vi "DAQ Input Handler.vi"(8 "error in (no error)":errorcluster, 11 "Message Queues out":T1) -> (0 "error out":errorcluster, 3 "Message Queue":refnum<queue>)   [LabVIEW 2014]
uses:
  support/Message Queue/All Message Queues.ctl
  support/Message Queue/Message Cluster.ctl
  Teszt/Teszt.ctl
  Teszt/Command.ctl
  Engine/Message.ctl
  Digital/Digital Input Cluster.ctl
  Digital/Digital Output Cluster.ctl
  <vilib>/Analysis/baseanly.llb/Mean (DBL).vi
  support/Message Queue/Enqueue Message (Single).vi
  <vilib>/Utility/error.llb/Error Cluster From Error Code.vi
  <vilib>/ErrorRing/Error Ring.xnode
  support/Message Queue/Message Queue.lvlib
  <vilib>/Analysis/NI_AALBase.lvlib
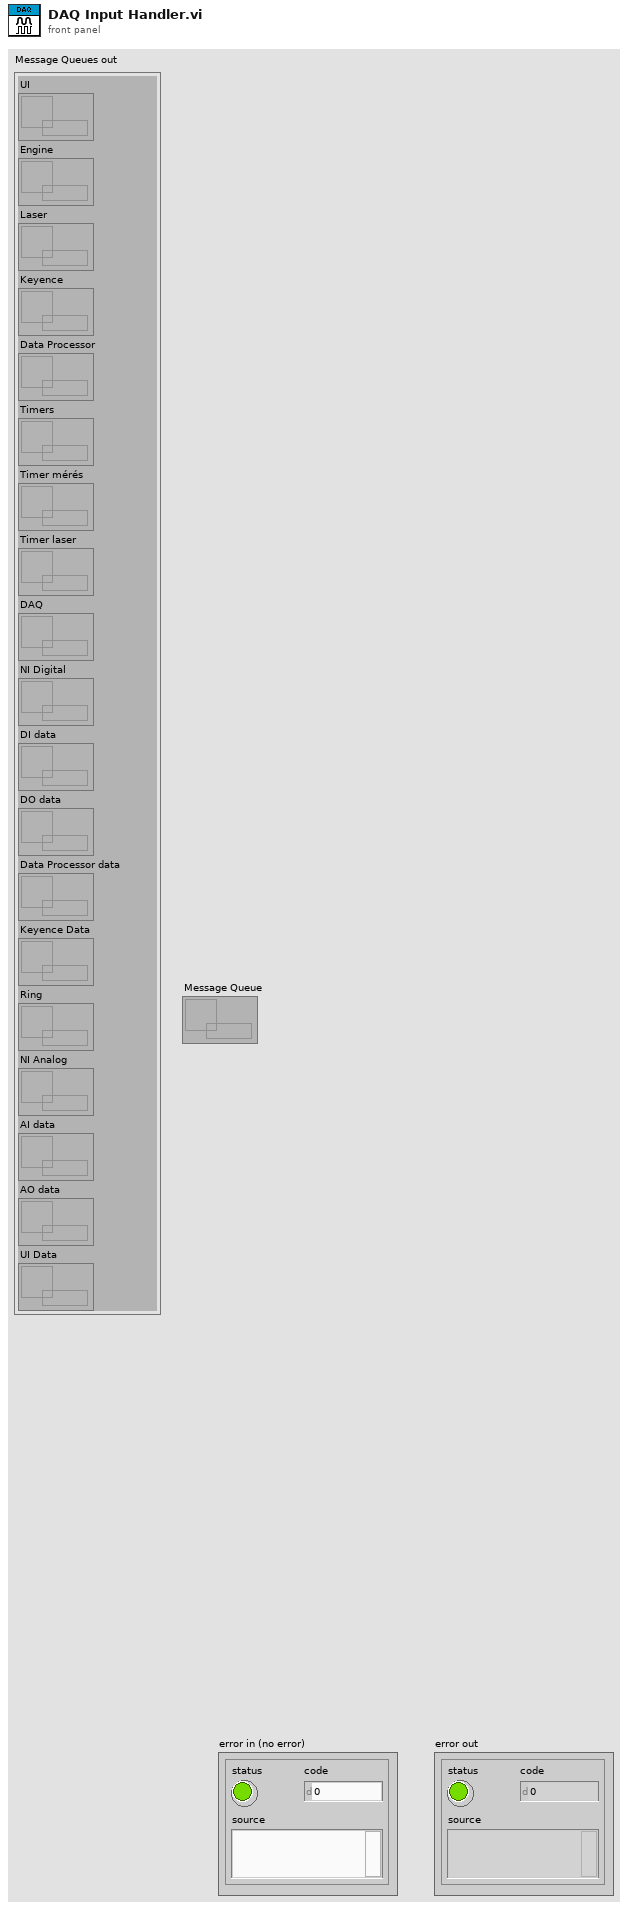
[diagram p1: front panel]
types:
  T1 = typedef "Message Queue.lvlib/All Message Queues.ctl" = cluster{"UI":refnum<queue>, "Engine":refnum<queue>, "Laser":refnum<queue>, "Keyence":refnum<queue>, "Data Processor":refnum<queue>, "Timers":refnum<queue>, "Timer mérés":refnum<queue>, "Timer laser":refnum<queue>, "DAQ":refnum<queue>, "NI Digital":refnum<queue>, "DI data":refnum<queue>, "DO data":refnum<queue>, "Data Processor data":refnum<queue>, "Keyence Data":refnum<queue>, "Ring":refnum<queue>, "NI Analog":refnum<queue>, "AI data":refnum<queue>, "AO data":refnum<queue>, "UI Data":refnum<queue>}
  T2 = typedef "Digital Output Cluster.ctl" = cluster{"PCIE-6321 OUT":cluster{"Izolációs relé":bool, "B oldal relé (nincs használva)":bool, "48V relé":bool, "Elszívás KI":bool, "Bördelezés teszt":bool, "Gyûrû megnyomás":bool, "Termék rögzítés":bool, "R mérés relé":bool, "200mA relé":bool, "NTC mérés relé":bool, "Levegõ BE":bool}}
  T3 = typedef "Digital Input Cluster.ctl" = cluster{"PCIE-6321 IN":cluster{"Termék bördelezve":bool, "Izolációs relék OK":bool, "Rézgyûrû a terméken":bool, "Termék rögzítve":bool, "Termék a gyûrûzõben":bool, "Rézgyûrû behelyezve":bool, "Rézgyûrû elengedve":bool, "Rézgyûrû megnyomva":bool, "Termék elengedve":bool, "Levegõ rendben":bool, "Termék jelen (táv)":bool, "Termék jelen (fém)":bool, "Selejt érzékelõ":bool}}
  T4 = typedef "Message.ctl" = cluster{"Thread ID":u16, "Callback":string, "Data":variant, "Error":errorcluster}
  T5 = typedef "Teszt.ctl" = cluster{"Thread ID":dbl, "Mérésszám":string, "Mérés/Utasítás":string, "Command":T6, "Min":string, "Max":string, "Aktív?":bool, "Log?":bool, "Kiértékelés":bool, "Etalon 1 exp":bool, "Etalon 2 exp":bool, "Etalon 3 exp":bool, "Etalon 4 exp":bool, "Etalon 5 exp":bool}
  T6 = typedef "Command.ctl" = cluster{"Parancs":string, "Paraméter 1":string, "Paraméter 2":string, "Paraméter 3":string, "Paraméter 4":string, "Paraméter 5":string, "Eredmény":string}
  T7 = cluster{"Termék bördelezve":bool, "Izolációs relék OK":bool, "Rézgyûrû a terméken":bool, "Termék rögzítve":bool, "Termék a gyûrûzõben":bool, "Rézgyûrû behelyezve":bool, "Rézgyûrû elengedve":bool, "Rézgyûrû megnyomva":bool, "Termék elengedve":bool, "Levegõ rendben":bool, "Termék jelen (táv)":bool, "Termék jelen (fém)":bool, "Selejt érzékelõ":bool}
  T8 = cluster{"Izolációs relé":bool, "B oldal relé (nincs használva)":bool, "48V relé":bool, "Elszívás KI":bool, "Bördelezés teszt":bool, "Gyûrû megnyomás":bool, "Termék rögzítés":bool, "R mérés relé":bool, "200mA relé":bool, "NTC mérés relé":bool, "Levegõ BE":bool}
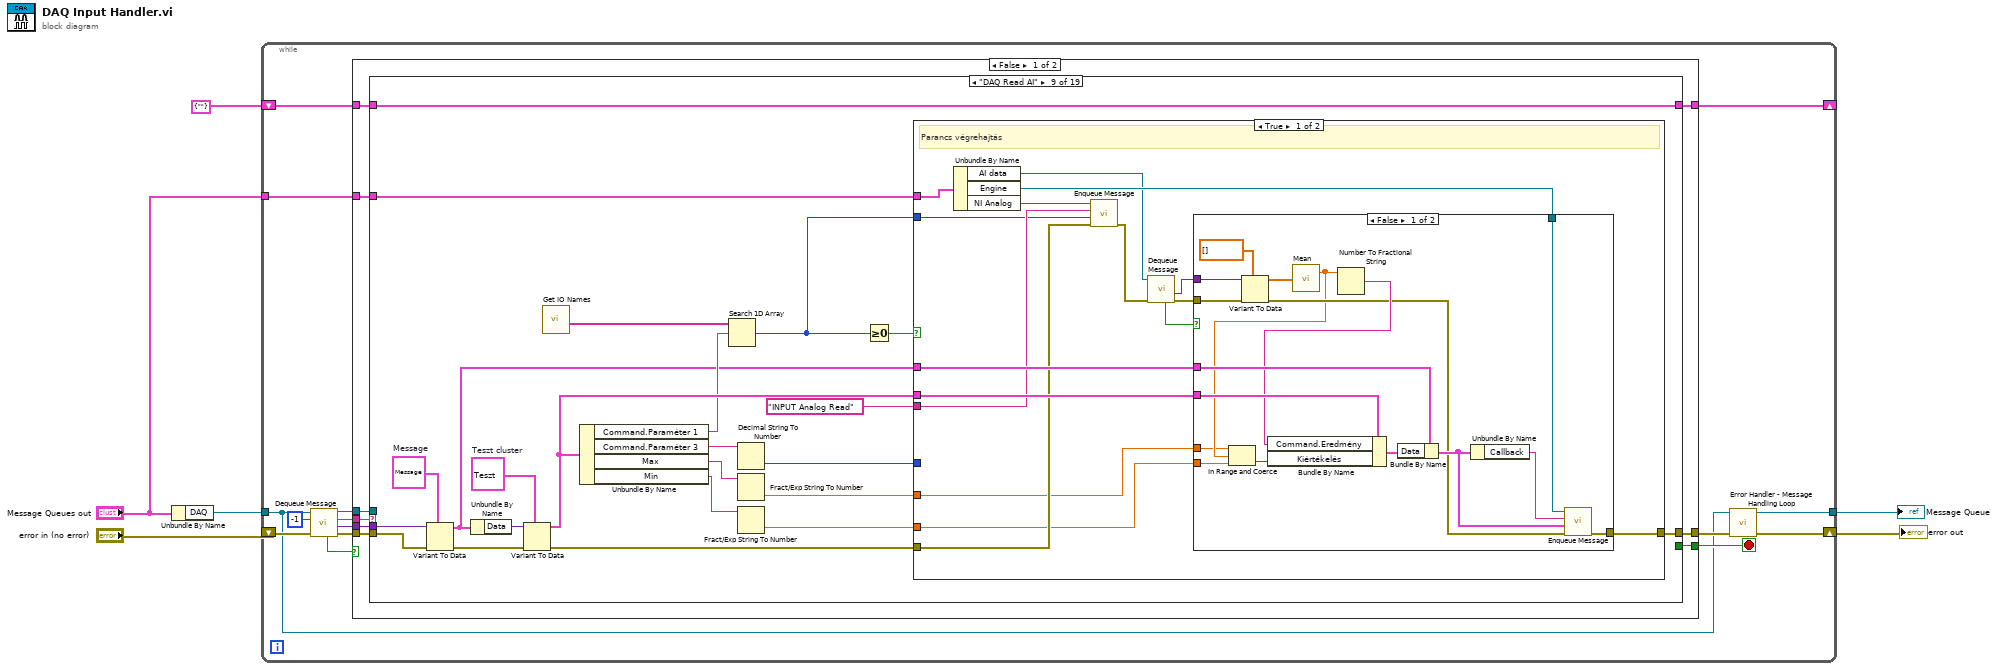
[diagram p0: block diagram]
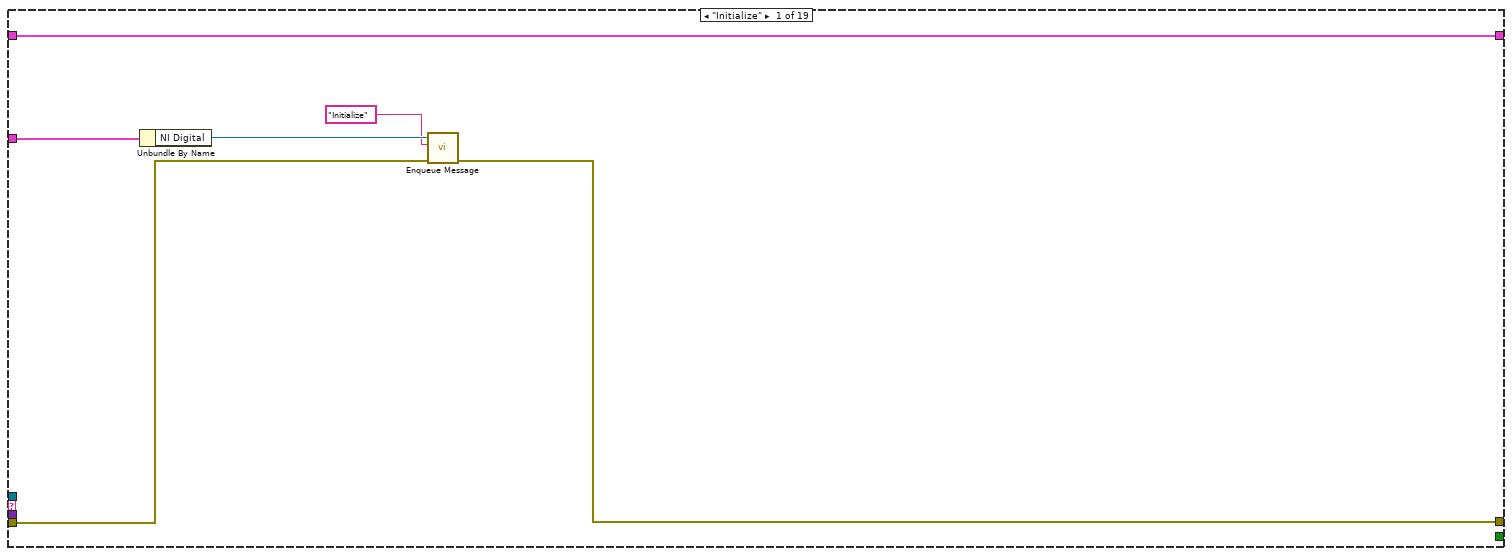
[diagram p2: hidden frame]
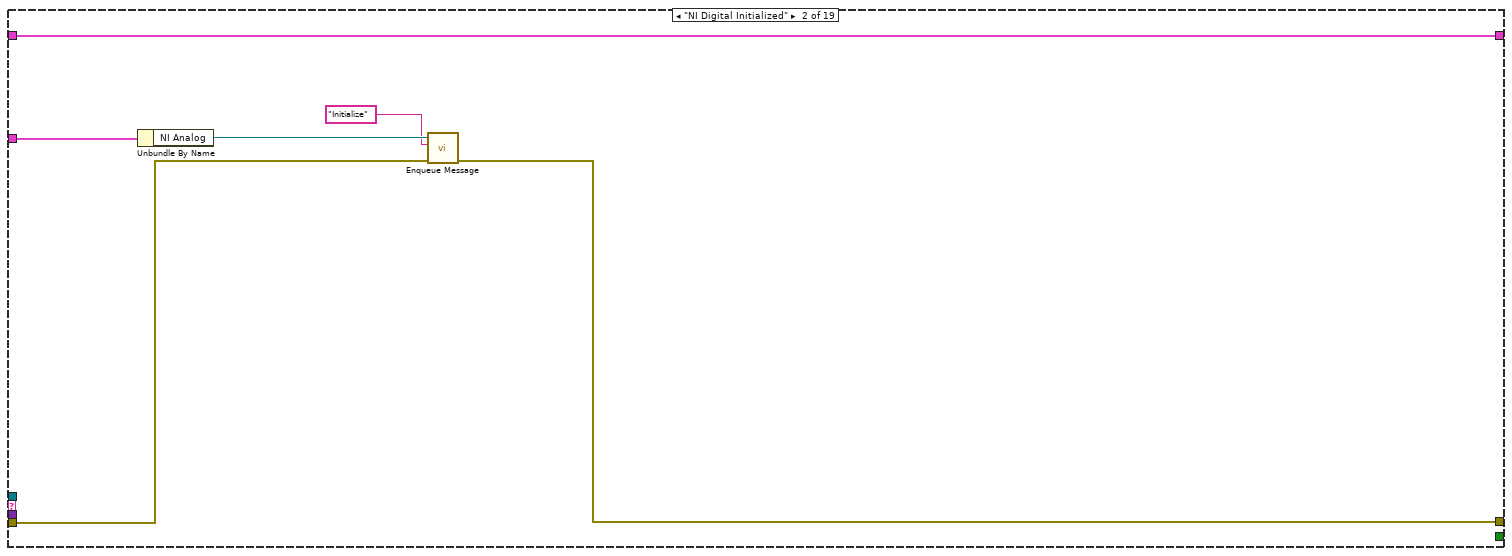
[diagram p3: hidden frame]
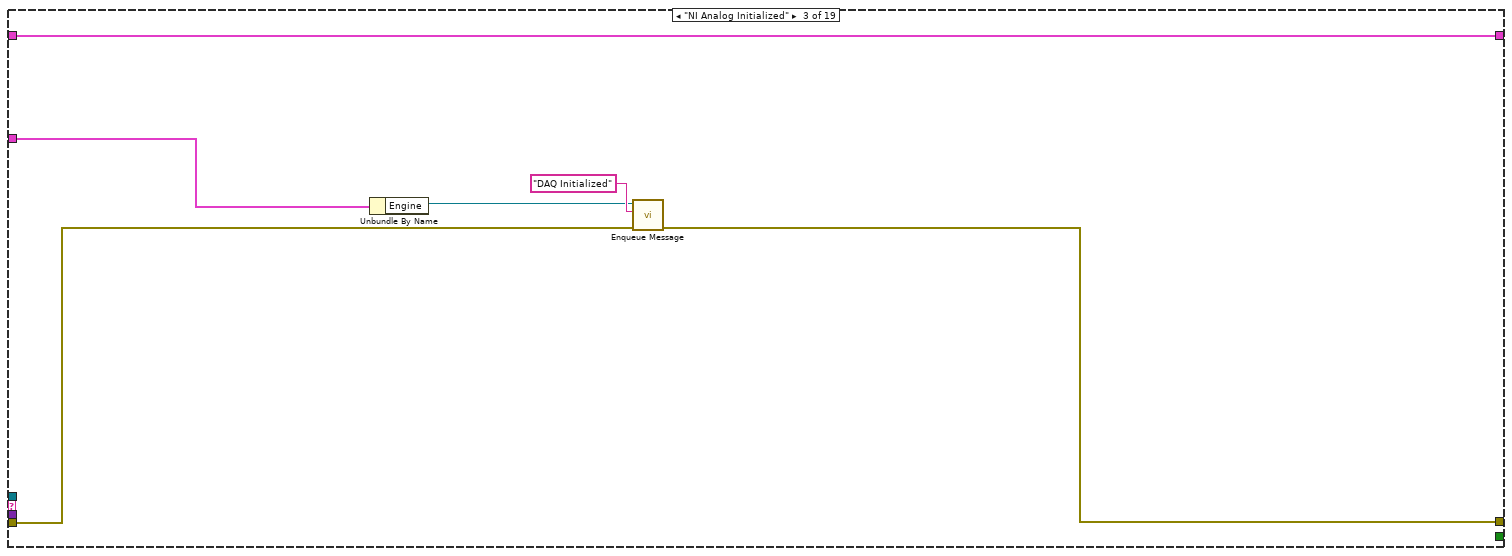
[diagram p4: hidden frame]
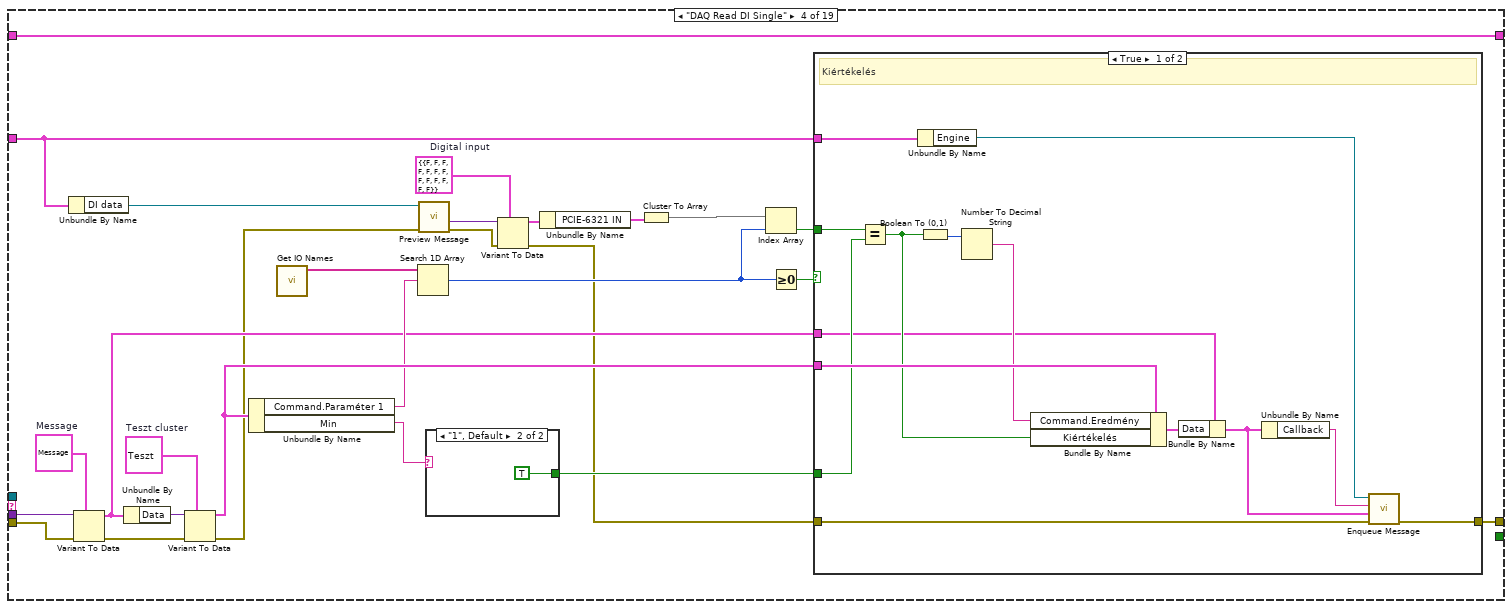
[diagram p5: hidden frame]
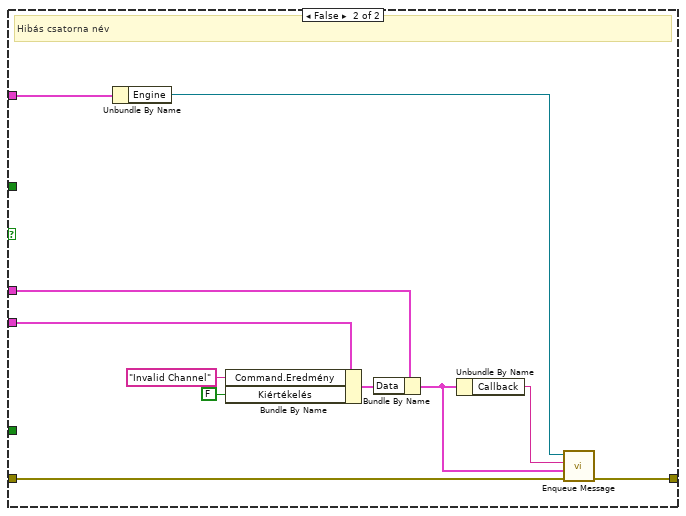
[diagram p6: hidden frame]
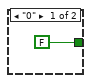
[diagram p7: hidden frame]
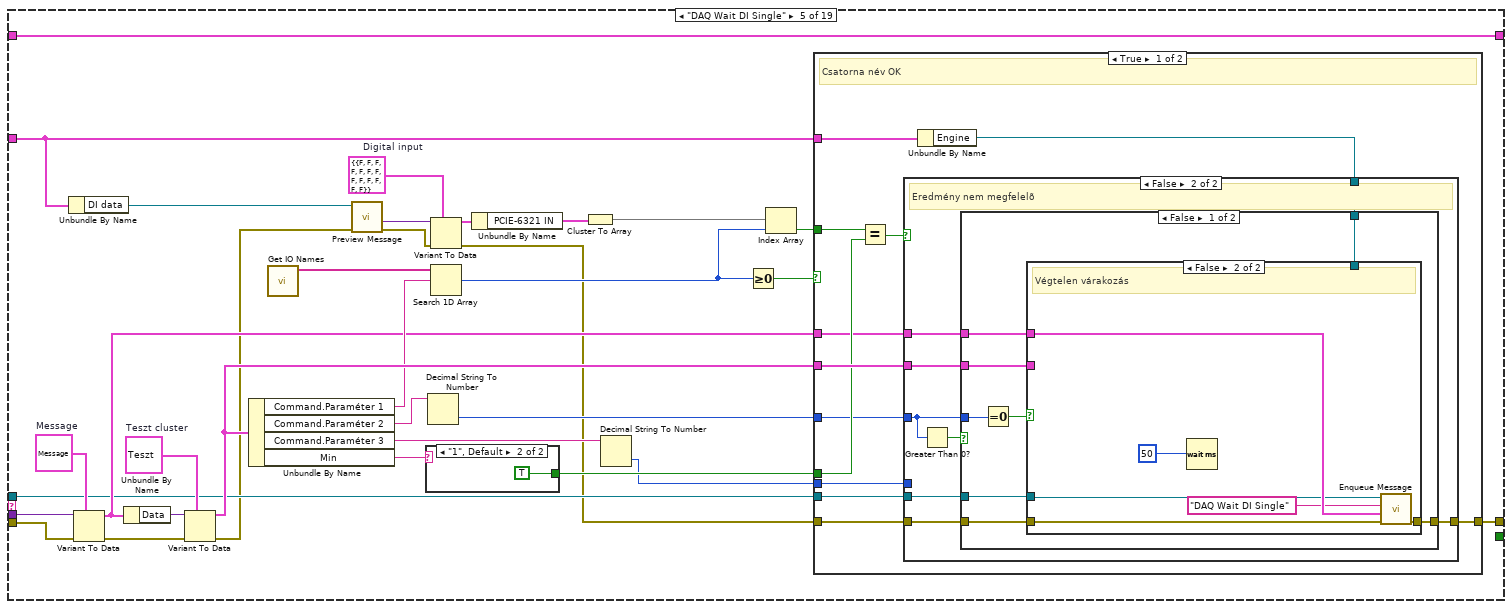
[diagram p8: hidden frame]
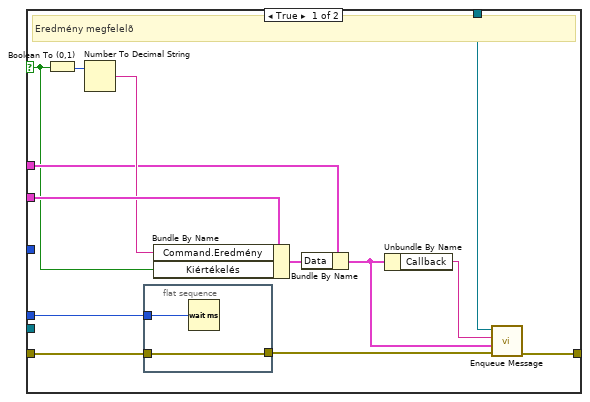
[diagram p9: hidden frame]
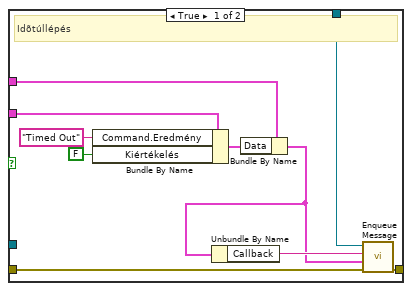
[diagram p10: hidden frame]
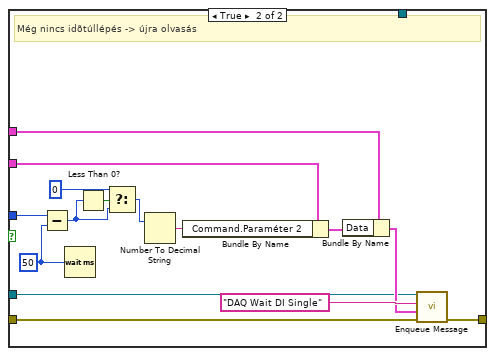
[diagram p11: hidden frame]
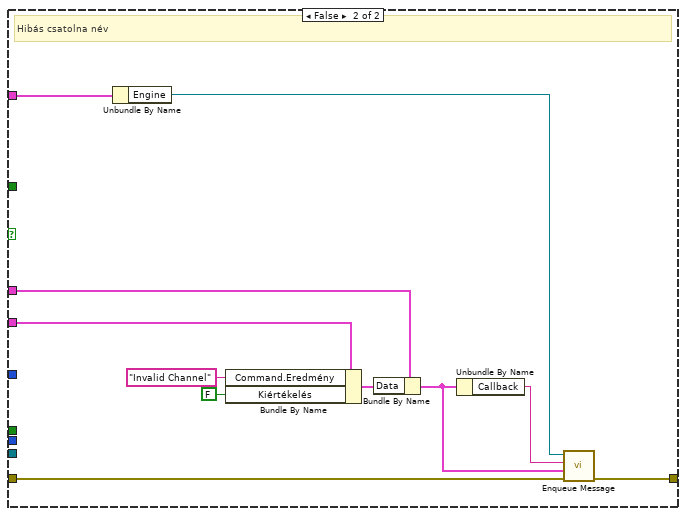
[diagram p12: hidden frame]
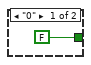
[diagram p13: hidden frame]
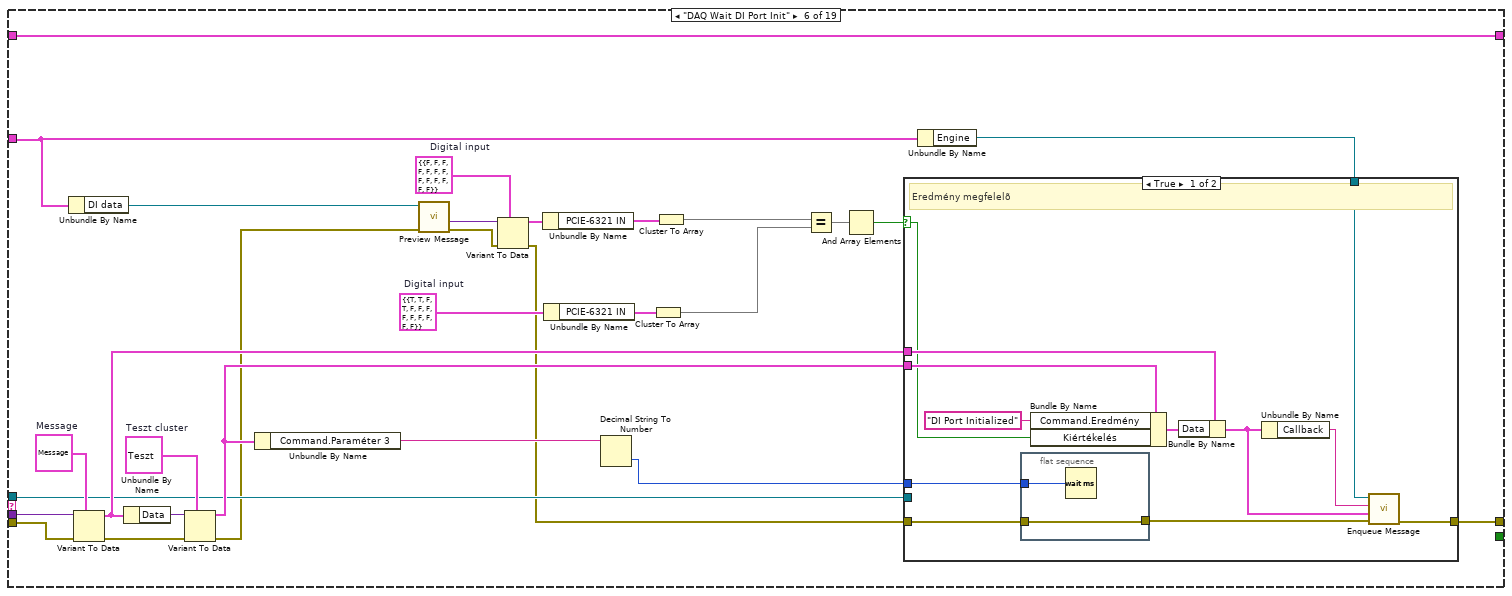
[diagram p14: hidden frame]
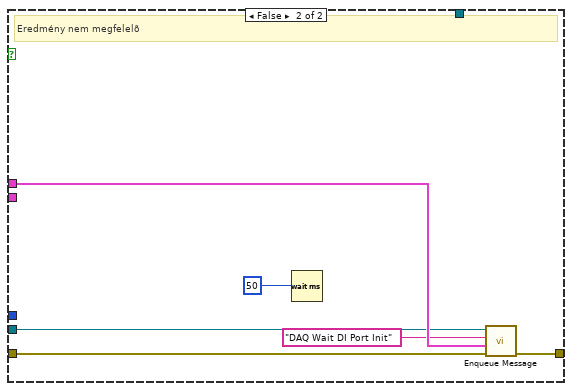
[diagram p15: hidden frame]
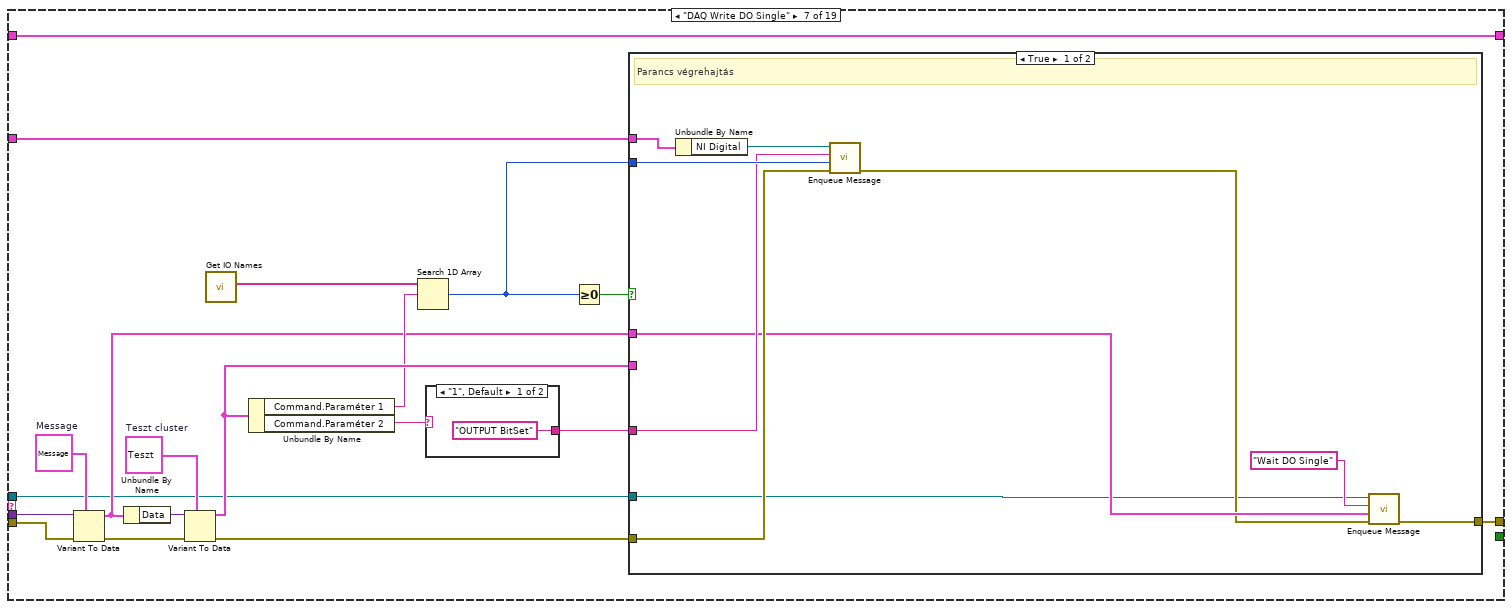
[diagram p16: hidden frame]
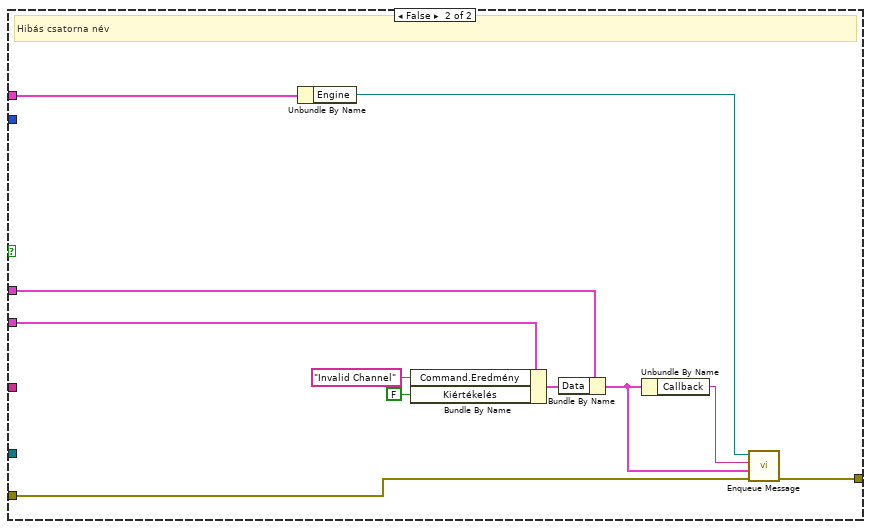
[diagram p17: hidden frame]
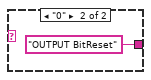
[diagram p18: hidden frame]
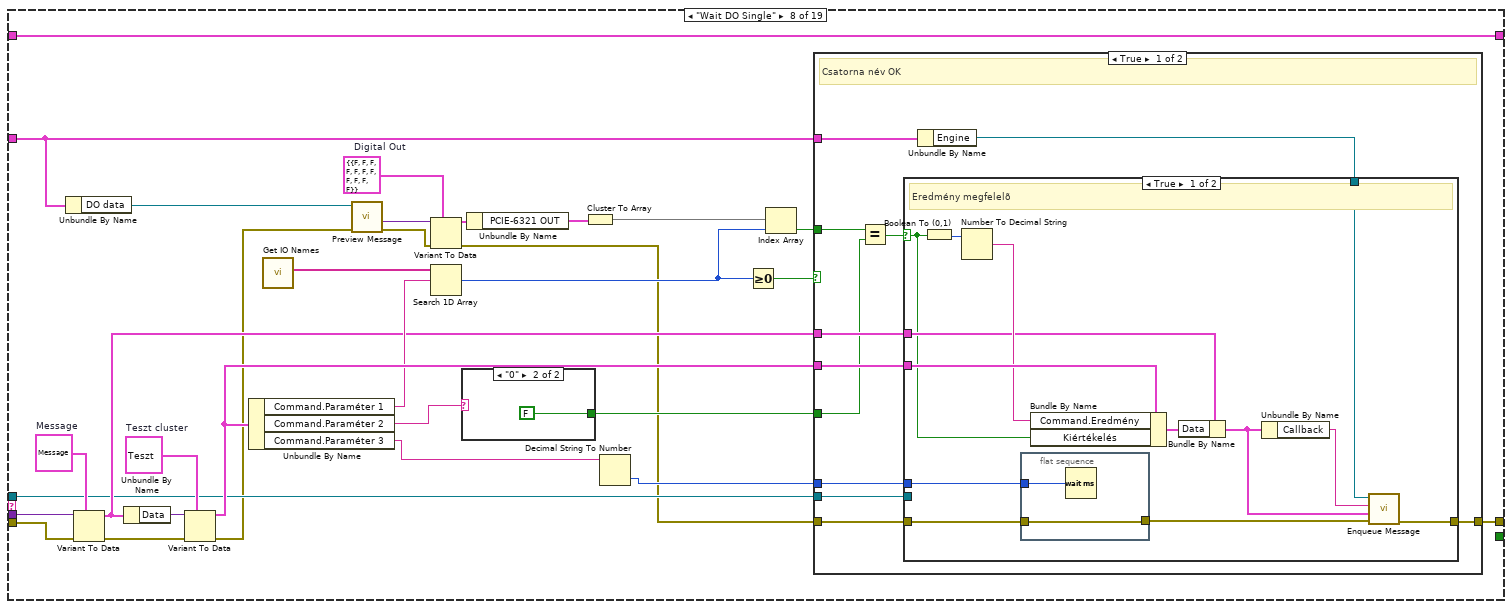
[diagram p19: hidden frame]
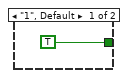
[diagram p20: hidden frame]
diagram:
  n1 = Unbundle By Name("Message Queues out") -> ("DAQ"=w3:refnum<queue>)
  n2 = while {
    tunnel: w3 -> [w7]
    shift-right: [w13] -> w6
    shift-left: "error in (no error)" -> [w21]
    tunnel: "Message Queues out" -> [w11]
    tunnel: [w10] -> w4
    shift-right: [w8] -> _
    shift-left: cluster{"Enabled Connectors":string} {"Enabled Connectors"=""} -> [w9]
    stop <- w17 stop-if-true
    n3 = call "Dequeue Message.vi"("error in (no error)"=w21, "timeout in ms (-1)"=-1, "Message Queue"=w7) -> ("error out"=w19:errorcluster, "Message Data"=w14:variant, "Message"=w20:string, "dup Message Queue"=w18:refnum<queue>, "timed out?"=w15:bool)  [unwired: 4 in]
    n4 = case shown="False" w15 {
      tunnel: w20 -> [w30 _]
      tunnel: w19 -> [w29 w655]
      tunnel: w18 -> [w28 _]
      tunnel: [w27 FALSE] -> w17
      tunnel: [w26 w655] -> w12
      tunnel: w14 -> [w25 _]
      tunnel: w11 -> [w24 _]
      tunnel: w9 -> [w23 w653]
      tunnel: [w22 w653] -> w8
      frame False {
        n5 = case shown="\"DAQ Read AI\"" w30 {
          selector: w30 -> [_ _ _ _ _ _ _ _ _ _ _ _ _ _ _ _ _ _ w643]
          tunnel: w29 -> [w33 w39 w44 w71 w130 w246 w284 w338 w405 w481 w538 w568 w587 w608 w619 w624 w633 w642 _]
          tunnel: w28 -> [_ _ _ _ w107 w234 w271 w319 _ _ _ _ _ _ w618 w631 w636 w641 _]
          tunnel: [w32 w38 w48 w70 w129 w245 w283 w337 w404 w480 w537 w567 w586 w607 w617 w621 w637 w639 w644] -> w26
          tunnel: [_ _ _ _ _ _ _ _ _ _ _ _ _ _ _ _ _ TRUE _] -> w27
          tunnel: w25 -> [_ _ _ w68 w127 w243 w281 w335 w402 w478 w535 w565 w585 w606 _ w625 _ _ _]
          tunnel: w24 -> [w34 w40 w43 w53 w113 w236 w274 w322 w396 w472 w531 w562 w581 w602 _ w626 _ _ _]
          tunnel: w23 -> [w31 w37 w46 w66 w125 w242 w279 w333 w400 w476 w534 w564 w584 w605 w616 w630 w635 w638 w645]
          tunnel: [w31 w37 w46 w66 w125 w242 w279 w333 w400 w476 w534 w564 w584 w605 w616 w630 w635 w638 w645] -> w22
          frame "Initialize" {
            n6 = Unbundle By Name(w34) -> ("NI Digital"=w36:refnum<queue>)
            n7 = call-poly "Enqueue Message.vi"("error in (no error)"=w33, "Message"="Initialize", "Message Queue"=w36) -> ("error out"=w32:errorcluster)  [unwired: 7 in, 1 out]
          }
          frame "NI Digital Initialized" {
            n8 = Unbundle By Name(w40) -> ("NI Analog"=w42:refnum<queue>)
            n9 = call-poly "Enqueue Message.vi"("error in (no error)"=w39, "Message"="Initialize", "Message Queue"=w42) -> ("error out"=w38:errorcluster)  [unwired: 7 in, 1 out]
          }
          frame "NI Analog Initialized" {
            n10 = Unbundle By Name(w43) -> ("Engine"=w45:refnum<queue>)
            n11 = call-poly "Enqueue Message.vi"("error in (no error)"=w44, "Message"="DAQ Initialized", "Message Queue"=w45) -> ("error out"=w48:errorcluster)  [unwired: 7 in, 1 out]
          }
          frame "DAQ Read DI Single" {
            w65 = T3 {"PCIE-6321 IN"={"Termék bördelezve"=FALSE, "Izolációs relék OK"=FALSE, "Rézgyûrû a terméken"=FALSE, "Termék rögzítve"=FALSE, "Termék a gyûrûzõben"=FALSE, "Rézgyûrû behelyezve"=FALSE, "Rézgyûrû elengedve"=FALSE, "Rézgyûrû megnyomva"=FALSE, "Termék elengedve"=FALSE, "Levegõ rendben"=FALSE, "Termék jelen (táv)"=FALSE, "Termék jelen (fém)"=FALSE, "Selejt érzékelõ"=FALSE}}  # Digital input
            w72 = T4 {"Thread ID"=0, "Callback"="", "Data"=variant, "Error"={"status"=FALSE, "code"=0, "source"=""}}  # Message
            w75 = T5 {"Thread ID"=0.0, "Mérésszám"="", "Mérés/Utasítás"="", "Command"={"Parancs"="", "Paraméter 1"="", "Paraméter 2"="", "Paraméter 3"="", "Paraméter 4"="", "Paraméter 5"="", "Eredmény"=""}, "Min"="", "Max"="", "Aktív?"=FALSE, "Log?"=FALSE, "Kiértékelés"=FALSE, "Etalon 1 exp"=FALSE, "Etalon 2 exp"=FALSE, "Etalon 3 exp"=FALSE, "Etalon 4 exp"=FALSE, "Etalon 5 exp"=FALSE}  # Teszt cluster
            n12 = Unbundle By Name(w53) -> ("DI data"=w62:refnum<queue>)
            n13 = Variant To Data(error in=w71, type=w72, Variant=w68) -> (data=w54:T4, error out=w74:errorcluster)
            n14 = Unbundle By Name(w54) -> ("Data"=w73:variant)
            n15 = Variant To Data(error in=w74, type=w75, Variant=w73) -> (data=w69:T5, error out=w50:errorcluster)
            n16 = Unbundle By Name(w69) -> ("Command.Paraméter 1"=w67:string, "Min"=w55:string)
            n17 = call "Get IO Names.vi"() -> ("DI Names"=w52:string[])  [unwired: 8 in, 3 out]
            n18 = Search 1D Array(1D array=w52, element=w67) -> (index of element=w59:i32)  [unwired: 1 in]
            n19 = call "Preview Message.vi"("error in (no error)"=w50, "Message Queue"=w62) -> ("error out"=w63:errorcluster, "Message Data"=w64:variant)  [unwired: 5 in, 3 out]
            n20 = case shown="\"1\", Default" w55 {
              tunnel: [FALSE TRUE] -> w56
              frame "0" {
              }
              frame "1", Default {
              }
            }
            n21 = Variant To Data(error in=w63, type=w65, Variant=w64) -> (data=w60:T3, error out=w49:errorcluster)
            n22 = Unbundle By Name(w60) -> ("PCIE-6321 IN"=w61:T7)
            n23 = Cluster To Array(cluster=w61) -> (array=w51:bool[])
            n24 = Index Array(array=w51, index=w59) -> (element=w57:bool)
            n25 = Greater Or Equal To 0?(x=w59) -> (x >= 0?=w58:bool)
            n26 = case shown="True" w58 {
              tunnel: w49 -> [w89 w100]
              tunnel: [w88 w99] -> w70
              tunnel: w69 -> [w87 w98]
              tunnel: w57 -> [w86 _]
              tunnel: w56 -> [w85 _]
              tunnel: w54 -> [w80 w96]
              tunnel: w53 -> [w77 w93]
              frame True {
                # "Kiértékelés"
                n27 = Equal?(x=w86, y=w85) -> (x = y?=w81:bool)
                n28 = Unbundle By Name(w77) -> ("Engine"=w76:refnum<queue>)
                n29 = Boolean To (0,1)(Boolean=w81) -> (0, 1=w83:i16)
                n30 = Number To Decimal String(number=w83) -> (decimal integer string=w82:string)  [unwired: 1 in]
                n31 = Bundle By Name(cluster=w87, "Command.Eredmény"=w82, "Kiértékelés"=w81) -> (w84:T5)
                n32 = Bundle By Name(cluster=w80, "Data"=w84) -> (w78:T4)
                n33 = Unbundle By Name(w78) -> ("Callback"=w79:string)
                n34 = call-poly "Enqueue Message.vi"("error in (no error)"=w89, "Message Data"=w78, "Message"=w79, "Message Queue"=w76) -> ("error out"=w88:errorcluster)  [unwired: 6 in, 1 out]
              }
              frame False {
                # "Hibás csatorna név"
                n35 = Unbundle By Name(w93) -> ("Engine"=w92:refnum<queue>)
                n36 = Bundle By Name(cluster=w98, "Command.Eredmény"="Invalid Channel", "Kiértékelés"=FALSE) -> (w97:T5)
                n37 = Bundle By Name(cluster=w96, "Data"=w97) -> (w94:T4)
                n38 = Unbundle By Name(w94) -> ("Callback"=w95:string)
                n39 = call-poly "Enqueue Message.vi"("error in (no error)"=w100, "Message Data"=w94, "Message"=w95, "Message Queue"=w92) -> ("error out"=w99:errorcluster)  [unwired: 6 in, 1 out]
              }
            }
          }
          frame "DAQ Wait DI Single" {
            w124 = T3 {"PCIE-6321 IN"={"Termék bördelezve"=FALSE, "Izolációs relék OK"=FALSE, "Rézgyûrû a terméken"=FALSE, "Termék rögzítve"=FALSE, "Termék a gyûrûzõben"=FALSE, "Rézgyûrû behelyezve"=FALSE, "Rézgyûrû elengedve"=FALSE, "Rézgyûrû megnyomva"=FALSE, "Termék elengedve"=FALSE, "Levegõ rendben"=FALSE, "Termék jelen (táv)"=FALSE, "Termék jelen (fém)"=FALSE, "Selejt érzékelõ"=FALSE}}  # Digital input
            w131 = T4 {"Thread ID"=0, "Callback"="", "Data"=variant, "Error"={"status"=FALSE, "code"=0, "source"=""}}  # Message
            w134 = T5 {"Thread ID"=0.0, "Mérésszám"="", "Mérés/Utasítás"="", "Command"={"Parancs"="", "Paraméter 1"="", "Paraméter 2"="", "Paraméter 3"="", "Paraméter 4"="", "Paraméter 5"="", "Eredmény"=""}, "Min"="", "Max"="", "Aktív?"=FALSE, "Log?"=FALSE, "Kiértékelés"=FALSE, "Etalon 1 exp"=FALSE, "Etalon 2 exp"=FALSE, "Etalon 3 exp"=FALSE, "Etalon 4 exp"=FALSE, "Etalon 5 exp"=FALSE}  # Teszt cluster
            n40 = Unbundle By Name(w113) -> ("DI data"=w121:refnum<queue>)
            n41 = Variant To Data(error in=w130, type=w131, Variant=w127) -> (data=w114:T4, error out=w133:errorcluster)
            n42 = Unbundle By Name(w114) -> ("Data"=w132:variant)
            n43 = Variant To Data(error in=w133, type=w134, Variant=w132) -> (data=w128:T5, error out=w104:errorcluster)
            n44 = Unbundle By Name(w128) -> ("Command.Paraméter 1"=w126:string, "Command.Paraméter 2"=w112:string, "Command.Paraméter 3"=w109:string, "Min"=w110:string)
            n45 = call "Get IO Names.vi"() -> ("DI Names"=w106:string[])  [unwired: 8 in, 3 out]
            n46 = call "Preview Message.vi"("error in (no error)"=w104, "Message Queue"=w121) -> ("error out"=w122:errorcluster, "Message Data"=w123:variant)  [unwired: 5 in, 3 out]
            n47 = case shown="\"1\", Default" w110 {
              tunnel: [FALSE TRUE] -> w115
              frame "0" {
              }
              frame "1", Default {
              }
            }
            n48 = Decimal String To Number(string=w112) -> (number=w111:i32)  [unwired: 2 in, 1 out]
            n49 = Variant To Data(error in=w122, type=w124, Variant=w123) -> (data=w119:T3, error out=w103:errorcluster)
            n50 = Search 1D Array(1D array=w106, element=w126) -> (index of element=w118:i32)  [unwired: 1 in]
            n51 = Unbundle By Name(w119) -> ("PCIE-6321 IN"=w120:T7)
            n52 = Cluster To Array(cluster=w120) -> (array=w105:bool[])
            n53 = Decimal String To Number(string=w109) -> (number=w108:i32)  [unwired: 2 in, 1 out]
            n54 = Greater Or Equal To 0?(x=w118) -> (x >= 0?=w117:bool)
            n55 = Index Array(array=w105, index=w118) -> (element=w116:bool)
            n56 = case shown="True" w117 {
              tunnel: w103 -> [w146 w219]
              tunnel: [w145 w218] -> w129
              tunnel: w128 -> [w144 w217]
              tunnel: w116 -> [w135 _]
              tunnel: w115 -> [w143 _]
              tunnel: w114 -> [w142 w215]
              tunnel: w113 -> [w141 w212]
              tunnel: w111 -> [w138 _]
              tunnel: w108 -> [w137 _]
              tunnel: w107 -> [w136 _]
              frame True {
                # "Csatorna név OK"
                n57 = Equal?(x=w135, y=w143) -> (x = y?=w139:bool)
                n58 = Unbundle By Name(w141) -> ("Engine"=w140:refnum<queue>)
                n59 = case shown="False" w139 {
                  selector: w139 -> [w150 _]
                  tunnel: w146 -> [w149 w169]
                  tunnel: [w159 w168] -> w145
                  tunnel: w144 -> [w158 w166]
                  tunnel: w142 -> [w154 w165]
                  tunnel: w140 -> [w151 w167]
                  tunnel: w138 -> [_ w164]
                  tunnel: w137 -> [w147 _]
                  tunnel: w136 -> [_ w162]
                  frame True {
                    # "Eredmény megfelelõ"
                    n60 = Boolean To (0,1)(Boolean=w150) -> (0, 1=w156:i16)
                    n61 = Number To Decimal String(number=w156) -> (decimal integer string=w155:string)  [unwired: 1 in]
                    n62 = flat-sequence {
                      tunnel: w147 -> [w161]
                      tunnel: [w160] -> w148
                      tunnel: w149 -> [w160]
                      frame #0 {
                        n63 = Wait (ms)(milliseconds to wait=w161) -> ()  [unwired: 1 out]
                      }
                    }
                    n64 = Bundle By Name(cluster=w158, "Command.Eredmény"=w155, "Kiértékelés"=w150) -> (w157:T5)
                    n65 = Bundle By Name(cluster=w154, "Data"=w157) -> (w152:T4)
                    n66 = Unbundle By Name(w152) -> ("Callback"=w153:string)
                    n67 = call-poly "Enqueue Message.vi"("error in (no error)"=w148, "Message Data"=w152, "Message"=w153, "Message Queue"=w151) -> ("error out"=w159:errorcluster)  [unwired: 6 in, 1 out]
                  }
                  frame False {
                    # "Eredmény nem megfelelõ"
                    n68 = Greater Than 0?(x=w164) -> (x > 0?=w163:bool)
                    n69 = case shown="False" w163 {
                      tunnel: w169 -> [w174 w208]
                      tunnel: [w175 w207] -> w168
                      tunnel: w167 -> [w173 _]
                      tunnel: w164 -> [w172 w205]
                      tunnel: w166 -> [w177 w203]
                      tunnel: w165 -> [w176 w201]
                      tunnel: w162 -> [w170 w194]
                      frame False {
                        n70 = Equal To 0?(x=w172) -> (x = 0?=w171:bool)
                        n71 = case shown="False" w171 {
                          tunnel: w177 -> [w184 _]
                          tunnel: w176 -> [w183 w191]
                          tunnel: [w182 w193] -> w175
                          tunnel: w174 -> [w181 w192]
                          tunnel: w173 -> [w180 _]
                          tunnel: w170 -> [_ w188]
                          frame True {
                            # "Idõtúllépés"
                            n72 = Bundle By Name(cluster=w184, "Command.Eredmény"="Timed Out", "Kiértékelés"=FALSE) -> (w187:T5)
                            n73 = Bundle By Name(cluster=w183, "Data"=w187) -> (w178:T4)
                            n74 = Unbundle By Name(w178) -> ("Callback"=w179:string)
                            n75 = call-poly "Enqueue Message.vi"("error in (no error)"=w181, "Message Data"=w178, "Message"=w179, "Message Queue"=w180) -> ("error out"=w182:errorcluster)  [unwired: 6 in, 1 out]
                          }
                          frame False {
                            # "Végtelen várakozás"
                            n76 = Wait (ms)(milliseconds to wait=50) -> ()  [unwired: 1 out]
                            n77 = call-poly "Enqueue Message.vi"("error in (no error)"=w192, "Message Data"=w191, "Message"="DAQ Wait DI Single", "Message Queue"=w188) -> ("error out"=w193:errorcluster)  [unwired: 6 in, 1 out]
                          }
                        }
                      }
                      frame True {
                        w204 = 50 ("milliseconds to wait")
                        # "Még nincs idõtúllépés -> újra olvasás"
                        n78 = Subtract(x=w205, y=w204) -> (x-y=w197:i32)
                        n79 = Wait (ms)(milliseconds to wait=w204) -> ()  [unwired: 1 out]
                        n80 = Less Than 0?(x=w197) -> (x < 0?=w198:bool)
                        n81 = Select(t=0, s=w198, f=w197) -> (s? t:f=w195:i32)
                        n82 = Number To Decimal String(number=w195) -> (decimal integer string=w202:string)  [unwired: 1 in]
                        n83 = Bundle By Name(cluster=w203, "Command.Paraméter 2"=w202) -> (w200:T5)
                        n84 = Bundle By Name(cluster=w201, "Data"=w200) -> (w199:T4)
                        n85 = call-poly "Enqueue Message.vi"("error in (no error)"=w208, "Message Data"=w199, "Message"="DAQ Wait DI Single", "Message Queue"=w194) -> ("error out"=w207:errorcluster)  [unwired: 6 in, 1 out]
                      }
                    }
                  }
                }
              }
              frame False {
                # "Hibás csatolna név"
                n86 = Unbundle By Name(w212) -> ("Engine"=w211:refnum<queue>)
                n87 = Bundle By Name(cluster=w217, "Command.Eredmény"="Invalid Channel", "Kiértékelés"=FALSE) -> (w216:T5)
                n88 = Bundle By Name(cluster=w215, "Data"=w216) -> (w213:T4)
                n89 = Unbundle By Name(w213) -> ("Callback"=w214:string)
                n90 = call-poly "Enqueue Message.vi"("error in (no error)"=w219, "Message Data"=w213, "Message"=w214, "Message Queue"=w211) -> ("error out"=w218:errorcluster)  [unwired: 6 in, 1 out]
              }
            }
          }
          frame "DAQ Wait DI Port Init" {
            w230 = T3 {"PCIE-6321 IN"={"Termék bördelezve"=TRUE, "Izolációs relék OK"=TRUE, "Rézgyûrû a terméken"=FALSE, "Termék rögzítve"=TRUE, "Termék a gyûrûzõben"=FALSE, "Rézgyûrû behelyezve"=FALSE, "Rézgyûrû elengedve"=FALSE, "Rézgyûrû megnyomva"=FALSE, "Termék elengedve"=FALSE, "Levegõ rendben"=FALSE, "Termék jelen (táv)"=FALSE, "Termék jelen (fém)"=FALSE, "Selejt érzékelõ"=FALSE}}  # Digital input
            w241 = T3 {"PCIE-6321 IN"={"Termék bördelezve"=FALSE, "Izolációs relék OK"=FALSE, "Rézgyûrû a terméken"=FALSE, "Termék rögzítve"=FALSE, "Termék a gyûrûzõben"=FALSE, "Rézgyûrû behelyezve"=FALSE, "Rézgyûrû elengedve"=FALSE, "Rézgyûrû megnyomva"=FALSE, "Termék elengedve"=FALSE, "Levegõ rendben"=FALSE, "Termék jelen (táv)"=FALSE, "Termék jelen (fém)"=FALSE, "Selejt érzékelõ"=FALSE}}  # Digital input
            w247 = T4 {"Thread ID"=0, "Callback"="", "Data"=variant, "Error"={"status"=FALSE, "code"=0, "source"=""}}  # Message
            w250 = T5 {"Thread ID"=0.0, "Mérésszám"="", "Mérés/Utasítás"="", "Command"={"Parancs"="", "Paraméter 1"="", "Paraméter 2"="", "Paraméter 3"="", "Paraméter 4"="", "Paraméter 5"="", "Eredmény"=""}, "Min"="", "Max"="", "Aktív?"=FALSE, "Log?"=FALSE, "Kiértékelés"=FALSE, "Etalon 1 exp"=FALSE, "Etalon 2 exp"=FALSE, "Etalon 3 exp"=FALSE, "Etalon 4 exp"=FALSE, "Etalon 5 exp"=FALSE}  # Teszt cluster
            n91 = Unbundle By Name(w236) -> ("DI data"=w238:refnum<queue>)
            n92 = Variant To Data(error in=w246, type=w247, Variant=w243) -> (data=w237:T4, error out=w249:errorcluster)
            n93 = Unbundle By Name(w237) -> ("Data"=w248:variant)
            n94 = Variant To Data(error in=w249, type=w250, Variant=w248) -> (data=w244:T5, error out=w223:errorcluster)
            n95 = Unbundle By Name(w244) -> ("Command.Paraméter 3"=w227:string)
            n96 = call "Preview Message.vi"("error in (no error)"=w223, "Message Queue"=w238) -> ("error out"=w239:errorcluster, "Message Data"=w240:variant)  [unwired: 5 in, 3 out]
            n97 = Variant To Data(error in=w239, type=w241, Variant=w240) -> (data=w231:T3, error out=w222:errorcluster)
            n98 = Unbundle By Name(w231) -> ("PCIE-6321 IN"=w232:T7)
            n99 = Unbundle By Name(w230) -> ("PCIE-6321 IN"=w226:T7)
            n100 = Decimal String To Number(string=w227) -> (number=w235:i32)  [unwired: 2 in, 1 out]
            n101 = Cluster To Array(cluster=w226) -> (array=w224:bool[])
            n102 = Cluster To Array(cluster=w232) -> (array=w225:bool[])
            n103 = Equal?(x=w225, y=w224) -> (x = y?=w229:bool[])
            n104 = And Array Elements(Boolean array=w229) -> (logical AND=w228:bool)
            n105 = Unbundle By Name(w236) -> ("Engine"=w233:refnum<queue>)
            n106 = case shown="True" w228 {
              selector: w228 -> [w255 _]
              tunnel: w222 -> [w254 w270]
              tunnel: [w262 w269] -> w245
              tunnel: w244 -> [w261 _]
              tunnel: w237 -> [w259 w268]
              tunnel: w233 -> [w256 _]
              tunnel: w235 -> [w252 _]
              tunnel: w234 -> [_ w267]
              frame True {
                # "Eredmény megfelelõ"
                n107 = flat-sequence {
                  tunnel: w252 -> [w264]
                  tunnel: [w263] -> w253
                  tunnel: w254 -> [w263]
                  frame #0 {
                    n108 = Wait (ms)(milliseconds to wait=w264) -> ()  [unwired: 1 out]
                  }
                }
                n109 = Bundle By Name(cluster=w261, "Command.Eredmény"="DI Port Initialized", "Kiértékelés"=w255) -> (w260:T5)
                n110 = Bundle By Name(cluster=w259, "Data"=w260) -> (w257:T4)
                n111 = Unbundle By Name(w257) -> ("Callback"=w258:string)
                n112 = call-poly "Enqueue Message.vi"("error in (no error)"=w253, "Message Data"=w257, "Message"=w258, "Message Queue"=w256) -> ("error out"=w262:errorcluster)  [unwired: 6 in, 1 out]
              }
              frame False {
                # "Eredmény nem megfelelõ"
                n113 = Wait (ms)(milliseconds to wait=50) -> ()  [unwired: 1 out]
                n114 = call-poly "Enqueue Message.vi"("error in (no error)"=w270, "Message Data"=w268, "Message"="DAQ Wait DI Port Init", "Message Queue"=w267) -> ("error out"=w269:errorcluster)  [unwired: 6 in, 1 out]
              }
            }
          }
          frame "DAQ Write DO Single" {
            w285 = T4 {"Thread ID"=0, "Callback"="", "Data"=variant, "Error"={"status"=FALSE, "code"=0, "source"=""}}  # Message
            w288 = T5 {"Thread ID"=0.0, "Mérésszám"="", "Mérés/Utasítás"="", "Command"={"Parancs"="", "Paraméter 1"="", "Paraméter 2"="", "Paraméter 3"="", "Paraméter 4"="", "Paraméter 5"="", "Eredmény"=""}, "Min"="", "Max"="", "Aktív?"=FALSE, "Log?"=FALSE, "Kiértékelés"=FALSE, "Etalon 1 exp"=FALSE, "Etalon 2 exp"=FALSE, "Etalon 3 exp"=FALSE, "Etalon 4 exp"=FALSE, "Etalon 5 exp"=FALSE}  # Teszt cluster
            n115 = Variant To Data(error in=w284, type=w285, Variant=w281) -> (data=w276:T4, error out=w287:errorcluster)
            n116 = Unbundle By Name(w276) -> ("Data"=w286:variant)
            n117 = Variant To Data(error in=w287, type=w288, Variant=w286) -> (data=w282:T5, error out=w289:errorcluster)
            n118 = call "Get IO Names.vi"() -> ("DO Names"=w272:string[])  [unwired: 8 in, 3 out]
            n119 = Unbundle By Name(w282) -> ("Command.Paraméter 1"=w280:string, "Command.Paraméter 2"=w277:string)
            n120 = Search 1D Array(1D array=w272, element=w280) -> (index of element=w273:i32)  [unwired: 1 in]
            n121 = case shown="\"1\", Default" w277 {
              tunnel: ["OUTPUT BitSet" ("Message") "OUTPUT BitReset" ("Message")] -> w275
              frame "1", Default {
              }
              frame "0" {
              }
            }
            n122 = Greater Or Equal To 0?(x=w273) -> (x >= 0?=w278:bool)
            n123 = case shown="True" w278 {
              tunnel: w289 -> [w296 w310]
              tunnel: [w299 w309] -> w283
              tunnel: w282 -> [_ w308]
              tunnel: w276 -> [w292 w306]
              tunnel: w274 -> [w298 w303]
              tunnel: w273 -> [w295 _]
              tunnel: w275 -> [w294 _]
              tunnel: w271 -> [w290 _]
              frame True {
                # "Parancs végrehajtás"
                n124 = Unbundle By Name(w298) -> ("NI Digital"=w297:refnum<queue>)
                n125 = call-poly "Enqueue Message.vi"("error in (no error)"=w296, "Message Data"=w295, "Message"=w294, "Message Queue"=w297) -> ("error out"=w291:errorcluster)  [unwired: 6 in, 1 out]
                n126 = call-poly "Enqueue Message.vi"("error in (no error)"=w291, "Message Data"=w292, "Message"="Wait DO Single", "Message Queue"=w290) -> ("error out"=w299:errorcluster)  [unwired: 6 in, 1 out]
              }
              frame False {
                # "Hibás csatorna név"
                n127 = Unbundle By Name(w303) -> ("Engine"=w302:refnum<queue>)
                n128 = Bundle By Name(cluster=w308, "Command.Eredmény"="Invalid Channel", "Kiértékelés"=FALSE) -> (w307:T5)
                n129 = Bundle By Name(cluster=w306, "Data"=w307) -> (w304:T4)
                n130 = Unbundle By Name(w304) -> ("Callback"=w305:string)
                n131 = call-poly "Enqueue Message.vi"("error in (no error)"=w310, "Message Data"=w304, "Message"=w305, "Message Queue"=w302) -> ("error out"=w309:errorcluster)  [unwired: 6 in, 1 out]
              }
            }
          }
          frame "Wait DO Single" {
            w332 = T2 {"PCIE-6321 OUT"={"Izolációs relé"=FALSE, "B oldal relé (nincs használva)"=FALSE, "48V relé"=FALSE, "Elszívás KI"=FALSE, "Bördelezés teszt"=FALSE, "Gyûrû megnyomás"=FALSE, "Termék rögzítés"=FALSE, "R mérés relé"=FALSE, "200mA relé"=FALSE, "NTC mérés relé"=FALSE, "Levegõ BE"=FALSE}}  # Digital Out
            w339 = T4 {"Thread ID"=0, "Callback"="", "Data"=variant, "Error"={"status"=FALSE, "code"=0, "source"=""}}  # Message
            w342 = T5 {"Thread ID"=0.0, "Mérésszám"="", "Mérés/Utasítás"="", "Command"={"Parancs"="", "Paraméter 1"="", "Paraméter 2"="", "Paraméter 3"="", "Paraméter 4"="", "Paraméter 5"="", "Eredmény"=""}, "Min"="", "Max"="", "Aktív?"=FALSE, "Log?"=FALSE, "Kiértékelés"=FALSE, "Etalon 1 exp"=FALSE, "Etalon 2 exp"=FALSE, "Etalon 3 exp"=FALSE, "Etalon 4 exp"=FALSE, "Etalon 5 exp"=FALSE}  # Teszt cluster
            n132 = Unbundle By Name(w322) -> ("DO data"=w329:refnum<queue>)
            n133 = Variant To Data(error in=w338, type=w339, Variant=w335) -> (data=w323:T4, error out=w341:errorcluster)
            n134 = Unbundle By Name(w323) -> ("Data"=w340:variant)
            n135 = Variant To Data(error in=w341, type=w342, Variant=w340) -> (data=w336:T5, error out=w314:errorcluster)
            n136 = Unbundle By Name(w336) -> ("Command.Paraméter 1"=w334:string, "Command.Paraméter 2"=w316:string, "Command.Paraméter 3"=w321:string)
            n137 = call "Get IO Names.vi"() -> ("DO Names"=w317:string[])  [unwired: 8 in, 3 out]
            n138 = call "Preview Message.vi"("error in (no error)"=w314, "Message Queue"=w329) -> ("error out"=w330:errorcluster, "Message Data"=w331:variant)  [unwired: 5 in, 3 out]
            n139 = Variant To Data(error in=w330, type=w332, Variant=w331) -> (data=w327:T2, error out=w313:errorcluster)
            n140 = Search 1D Array(1D array=w317, element=w334) -> (index of element=w326:i32)  [unwired: 1 in]
            n141 = case shown="\"0\"" w316 {
              tunnel: [TRUE FALSE] -> w315
              frame "1", Default {
              }
              frame "0" {
              }
            }
            n142 = Unbundle By Name(w327) -> ("PCIE-6321 OUT"=w328:T8)
            n143 = Cluster To Array(cluster=w328) -> (array=w318:bool[])
            n144 = Decimal String To Number(string=w321) -> (number=w320:i32)  [unwired: 2 in, 1 out]
            n145 = Greater Or Equal To 0?(x=w326) -> (x >= 0?=w325:bool)
            n146 = Index Array(array=w318, index=w326) -> (element=w324:bool)
            n147 = case shown="True" w325 {
              tunnel: w313 -> [w355 w387]
              tunnel: [w354 w386] -> w337
              tunnel: w336 -> [w353 w385]
              tunnel: w324 -> [w346 _]
              tunnel: w323 -> [w352 w383]
              tunnel: w322 -> [w351 w380]
              tunnel: w320 -> [w348 _]
              tunnel: w319 -> [w347 _]
              tunnel: w315 -> [w345 _]
              frame True {
                # "Csatorna név OK"
                n148 = Equal?(x=w346, y=w345) -> (x = y?=w349:bool)
                n149 = Unbundle By Name(w351) -> ("Engine"=w350:refnum<queue>)
                n150 = case shown="True" w349 {
                  selector: w349 -> [w359 _]
                  tunnel: w355 -> [w358 w376]
                  tunnel: [w368 w375] -> w354
                  tunnel: w353 -> [w367 _]
                  tunnel: w352 -> [w363 w374]
                  tunnel: w350 -> [w360 _]
                  tunnel: w348 -> [w356 _]
                  tunnel: w347 -> [_ w373]
                  frame True {
                    # "Eredmény megfelelõ"
                    n151 = Boolean To (0,1)(Boolean=w359) -> (0, 1=w365:i16)
                    n152 = Number To Decimal String(number=w365) -> (decimal integer string=w364:string)  [unwired: 1 in]
                    n153 = flat-sequence {
                      tunnel: w356 -> [w370]
                      tunnel: [w369] -> w357
                      tunnel: w358 -> [w369]
                      frame #0 {
                        n154 = Wait (ms)(milliseconds to wait=w370) -> ()  [unwired: 1 out]
                      }
                    }
                    n155 = Bundle By Name(cluster=w367, "Command.Eredmény"=w364, "Kiértékelés"=w359) -> (w366:T5)
                    n156 = Bundle By Name(cluster=w363, "Data"=w366) -> (w361:T4)
                    n157 = Unbundle By Name(w361) -> ("Callback"=w362:string)
                    n158 = call-poly "Enqueue Message.vi"("error in (no error)"=w357, "Message Data"=w361, "Message"=w362, "Message Queue"=w360) -> ("error out"=w368:errorcluster)  [unwired: 6 in, 1 out]
                  }
                  frame False {
                    # "Eredmény nem megfelelõ"
                    n159 = Wait (ms)(milliseconds to wait=5) -> ()  [unwired: 1 out]
                    n160 = call-poly "Enqueue Message.vi"("error in (no error)"=w376, "Message Data"=w374, "Message"="Wait DO Single", "Message Queue"=w373) -> ("error out"=w375:errorcluster)  [unwired: 6 in, 1 out]
                  }
                }
              }
              frame False {
                # "Hibás csatolna név"
                n161 = Unbundle By Name(w380) -> ("Engine"=w379:refnum<queue>)
                n162 = Bundle By Name(cluster=w385, "Command.Eredmény"="Invalid Channel", "Kiértékelés"=FALSE) -> (w384:T5)
                n163 = Bundle By Name(cluster=w383, "Data"=w384) -> (w381:T4)
                n164 = Unbundle By Name(w381) -> ("Callback"=w382:string)
                n165 = call-poly "Enqueue Message.vi"("error in (no error)"=w387, "Message Data"=w381, "Message"=w382, "Message Queue"=w379) -> ("error out"=w386:errorcluster)  [unwired: 6 in, 1 out]
              }
            }
          }
          frame "DAQ Read AI" {
            w406 = T4 {"Thread ID"=0, "Callback"="", "Data"=variant, "Error"={"status"=FALSE, "code"=0, "source"=""}}  # Message
            w409 = T5 {"Thread ID"=0.0, "Mérésszám"="", "Mérés/Utasítás"="", "Command"={"Parancs"="", "Paraméter 1"="", "Paraméter 2"="", "Paraméter 3"="", "Paraméter 4"="", "Paraméter 5"="", "Eredmény"=""}, "Min"="", "Max"="", "Aktív?"=FALSE, "Log?"=FALSE, "Kiértékelés"=FALSE, "Etalon 1 exp"=FALSE, "Etalon 2 exp"=FALSE, "Etalon 3 exp"=FALSE, "Etalon 4 exp"=FALSE, "Etalon 5 exp"=FALSE}  # Teszt cluster
            n166 = Variant To Data(error in=w405, type=w406, Variant=w402) -> (data=w398:T4, error out=w408:errorcluster)
            n167 = Unbundle By Name(w398) -> ("Data"=w407:variant)
            n168 = Variant To Data(error in=w408, type=w409, Variant=w407) -> (data=w403:T5, error out=w410:errorcluster)
            n169 = call "Get IO Names.vi"() -> ("AI Names"=w393:string[])  [unwired: 8 in, 3 out]
            n170 = Unbundle By Name(w403) -> ("Command.Paraméter 1"=w401:string, "Command.Paraméter 3"=w395:string, "Max"=w391:string, "Min"=w390:string)
            n171 = Search 1D Array(1D array=w393, element=w401) -> (index of element=w392:i32)  [unwired: 1 in]
            n172 = Decimal String To Number(string=w395) -> (number=w394:i32)  [unwired: 2 in, 1 out]
            n173 = Fract/Exp String To Number(string=w391) -> (number=w389:dbl)  [unwired: 3 in, 1 out]
            n174 = Fract/Exp String To Number(string=w390) -> (number=w388:dbl)  [unwired: 3 in, 1 out]
            n175 = Greater Or Equal To 0?(x=w392) -> (x >= 0?=w399:bool)
            n176 = case shown="True" w399 {
              tunnel: w410 -> [w420 w464]
              tunnel: [w426 w463] -> w404
              tunnel: w403 -> [w425 w462]
              tunnel: w398 -> [w424 w460]
              tunnel: w396 -> [w423 w457]
              tunnel: w392 -> [w418 _]
              tunnel: "INPUT Analog Read" ("Message") -> [w419 _]
              tunnel: w394 -> [_ _]
              tunnel: w389 -> [w414 _]
              tunnel: w388 -> [w413 _]
              frame True {
                # "Parancs végrehajtás"
                n177 = Unbundle By Name(w423) -> ("AI data"=w416:refnum<queue>, "Engine"=w422:refnum<queue>, "NI Analog"=w421:refnum<queue>)
                n178 = call-poly "Enqueue Message.vi"("error in (no error)"=w420, "Message Data"=w418, "Message"=w419, "Message Queue"=w421) -> ("error out"=w415:errorcluster)  [unwired: 6 in, 1 out]
                n179 = call "Dequeue Message.vi"("error in (no error)"=w415, "Message Queue"=w416) -> ("error out"=w411:errorcluster, "Message Data"=w417:variant, "timed out?"=w412:bool)  [unwired: 5 in, 2 out]
                n180 = case shown="False" w412 {
                  tunnel: [w443 w449] -> w426
                  tunnel: w425 -> [w442 w447]
                  tunnel: w424 -> [w440 w448]
                  tunnel: w422 -> [w437 w445]
                  tunnel: w417 -> [w435 _]
                  tunnel: w414 -> [w429 _]
                  tunnel: w413 -> [w428 _]
                  tunnel: w411 -> [w427 w444]
                  frame False {
                    n181 = Variant To Data(error in=w427, type=dbl[] [], Variant=w435) -> (data=w434:dbl[], error out=w432:errorcluster)
                    n182 = call-poly <vilib>:"Mean.vi"("X"=w434) -> ("mean"=w430:dbl)  [unwired: 1 out]
                    n183 = In Range and Coerce(upper limit=w429, x=w430, lower limit=w428) -> (In Range?=w431:bool)  [unwired: 1 out]
                    n184 = Number To Fractional String(number=w430) -> (F-format string=w433:string)  [unwired: 3 in]
                    n185 = Bundle By Name(cluster=w442, "Command.Eredmény"=w433, "Kiértékelés"=w431) -> (w441:T5)
                    n186 = Bundle By Name(cluster=w440, "Data"=w441) -> (w438:T4)
                    n187 = Unbundle By Name(w438) -> ("Callback"=w439:string)
                    n188 = call-poly "Enqueue Message.vi"("error in (no error)"=w432, "Message Data"=w438, "Message"=w439, "Message Queue"=w437) -> ("error out"=w443:errorcluster)  [unwired: 6 in, 1 out]
                  }
                  frame True {
                    n189 = Bundle By Name(cluster=w447, "Command.Eredmény"="Timed Out", "Kiértékelés"=FALSE) -> (w450:T5)
                    n190 = Bundle By Name(cluster=w448, "Data"=w450) -> (w452:T4)
                    n191 = Unbundle By Name(w452) -> ("Callback"=w451:string)
                    n192 = call-poly "Enqueue Message.vi"("error in (no error)"=w444, "Message Data"=w452, "Message"=w451, "Message Queue"=w445) -> ("error out"=w449:errorcluster)  [unwired: 6 in, 1 out]
                  }
                }
              }
              frame False {
                # "Hibás csatorna név"
                n193 = Unbundle By Name(w457) -> ("Engine"=w456:refnum<queue>)
                n194 = Bundle By Name(cluster=w462, "Command.Eredmény"="Invalid Channel", "Kiértékelés"=FALSE) -> (w461:T5)
                n195 = Bundle By Name(cluster=w460, "Data"=w461) -> (w458:T4)
                n196 = Unbundle By Name(w458) -> ("Callback"=w459:string)
                n197 = call-poly "Enqueue Message.vi"("error in (no error)"=w464, "Message Data"=w458, "Message"=w459, "Message Queue"=w456) -> ("error out"=w463:errorcluster)  [unwired: 6 in, 1 out]
              }
            }
          }
          frame "DAQ Write AO" {
            w482 = T4 {"Thread ID"=0, "Callback"="", "Data"=variant, "Error"={"status"=FALSE, "code"=0, "source"=""}}  # Message
            w485 = T5 {"Thread ID"=0.0, "Mérésszám"="", "Mérés/Utasítás"="", "Command"={"Parancs"="", "Paraméter 1"="", "Paraméter 2"="", "Paraméter 3"="", "Paraméter 4"="", "Paraméter 5"="", "Eredmény"=""}, "Min"="", "Max"="", "Aktív?"=FALSE, "Log?"=FALSE, "Kiértékelés"=FALSE, "Etalon 1 exp"=FALSE, "Etalon 2 exp"=FALSE, "Etalon 3 exp"=FALSE, "Etalon 4 exp"=FALSE, "Etalon 5 exp"=FALSE}  # Teszt cluster
            n198 = Variant To Data(error in=w481, type=w482, Variant=w478) -> (data=w474:T4, error out=w484:errorcluster)
            n199 = Unbundle By Name(w474) -> ("Data"=w483:variant)
            n200 = Variant To Data(error in=w484, type=w485, Variant=w483) -> (data=w479:T5, error out=w486:errorcluster)
            n201 = call "Get IO Names.vi"() -> ("AO Names"=w468:string[])  [unwired: 8 in, 3 out]
            n202 = Unbundle By Name(w479) -> ("Command.Paraméter 1"=w477:string, "Command.Paraméter 2"=w467:string, "Command.Paraméter 3"=w470:string)
            n203 = Search 1D Array(1D array=w468, element=w477) -> (index of element=w471:i32)  [unwired: 1 in]
            n204 = Decimal String To Number(string=w470) -> (number=w469:i32)  [unwired: 2 in, 1 out]
            n205 = Decimal String To Number(string=w467) -> (number=w466:i32)  [unwired: 2 in, 1 out]
            n206 = To Double Precision Float(number=w466) -> (double precision float=w465:dbl)
            n207 = Greater Or Equal To 0?(x=w471) -> (x >= 0?=w475:bool)
            n208 = case shown="True" w475 {
              tunnel: w486 -> [w496 w518]
              tunnel: [w505 w517] -> w480
              tunnel: w479 -> [w504 w516]
              tunnel: w474 -> [w502 w514]
              tunnel: w472 -> [w499 w511]
              tunnel: w471 -> [w490 _]
              tunnel: "OUTPUT Analog Write" ("Message") -> [w495 _]
              tunnel: w469 -> [w493 _]
              tunnel: w467 -> [w487 _]
              tunnel: w465 -> [w488 _]
              frame True {
                # "Parancs végrehajtás"
                n209 = Unbundle By Name(w499) -> ("Engine"=w498:refnum<queue>, "NI Analog"=w497:refnum<queue>)
                n210 = Bundle("index of element"=w490, w488) -> (w489:cluster{"index of element":i32, dbl})  [unwired: 1 in]
                n211 = call-poly "Enqueue Message.vi"("error in (no error)"=w496, "Message Data"=w489, "Message"=w495, "Message Queue"=w497) -> ("error out"=w494:errorcluster)  [unwired: 6 in, 1 out]
                n212 = flat-sequence {
                  tunnel: w494 -> [w506]
                  tunnel: w493 -> [w507]
                  tunnel: [w506] -> w491
                  frame #0 {
                    n213 = Wait (ms)(milliseconds to wait=w507) -> ()  [unwired: 1 out]
                  }
                }
                n214 = Bundle By Name(cluster=w504, "Command.Eredmény"=w487, "Kiértékelés"=TRUE) -> (w503:T5)
                n215 = Bundle By Name(cluster=w502, "Data"=w503) -> (w500:T4)
                n216 = Unbundle By Name(w500) -> ("Callback"=w501:string)
                n217 = call-poly "Enqueue Message.vi"("error in (no error)"=w491, "Message Data"=w500, "Message"=w501, "Message Queue"=w498) -> ("error out"=w505:errorcluster)  [unwired: 6 in, 1 out]
              }
              frame False {
                # "Hibás csatorna név"
                n218 = Unbundle By Name(w511) -> ("Engine"=w510:refnum<queue>)
                n219 = Bundle By Name(cluster=w516, "Command.Eredmény"="Invalid Channel", "Kiértékelés"=FALSE) -> (w515:T5)
                n220 = Bundle By Name(cluster=w514, "Data"=w515) -> (w512:T4)
                n221 = Unbundle By Name(w512) -> ("Callback"=w513:string)
                n222 = call-poly "Enqueue Message.vi"("error in (no error)"=w518, "Message Data"=w512, "Message"=w513, "Message Queue"=w510) -> ("error out"=w517:errorcluster)  [unwired: 6 in, 1 out]
              }
            }
          }
          frame "DAQ dU Puffer" {
            w539 = T4 {"Thread ID"=0, "Callback"="", "Data"=variant, "Error"={"status"=FALSE, "code"=0, "source"=""}}  # Message
            w542 = T5 {"Thread ID"=0.0, "Mérésszám"="", "Mérés/Utasítás"="", "Command"={"Parancs"="", "Paraméter 1"="", "Paraméter 2"="", "Paraméter 3"="", "Paraméter 4"="", "Paraméter 5"="", "Eredmény"=""}, "Min"="", "Max"="", "Aktív?"=FALSE, "Log?"=FALSE, "Kiértékelés"=FALSE, "Etalon 1 exp"=FALSE, "Etalon 2 exp"=FALSE, "Etalon 3 exp"=FALSE, "Etalon 4 exp"=FALSE, "Etalon 5 exp"=FALSE}  # Teszt cluster
            n223 = Variant To Data(error in=w538, type=w539, Variant=w535) -> (data=w533:T4, error out=w541:errorcluster)
            n224 = Unbundle By Name(w533) -> ("Data"=w540:variant)
            n225 = Variant To Data(error in=w541, type=w542, Variant=w540) -> (data=w536:T5, error out=w543:errorcluster)
            n226 = Unbundle By Name(w536) -> ("Command.Paraméter 1"=w520:string, "Command.Paraméter 3"=w530:string)
            n227 = Decimal String To Number(string=w530) -> (number=w529:i32)  [unwired: 2 in, 1 out]
            n228 = case shown="\"Stop\"" w520 {
              tunnel: ["Delta U Puffer clear" ("Message") "Delta U Puffer start" ("Message") "Delta U Puffer stop" ("Message")] -> w532
              frame "Clear", Default {
              }
              frame "Start" {
              }
              frame "Stop" {
              }
            }
            n229 = Unbundle By Name(w531) -> ("Engine"=w525:refnum<queue>, "NI Analog"=w524:refnum<queue>)
            n230 = call-poly "Enqueue Message.vi"("error in (no error)"=w543, "Message"=w532, "Message Queue"=w524) -> ("error out"=w523:errorcluster)  [unwired: 7 in, 1 out]
            n231 = flat-sequence {
              tunnel: w523 -> [w547]
              tunnel: w529 -> [w548]
              tunnel: [w547] -> w521
              frame #0 {
                n232 = Wait (ms)(milliseconds to wait=w548) -> ()  [unwired: 1 out]
              }
            }
            n233 = Bundle By Name(cluster=w536, "Command.Eredmény"="Kész", "Kiértékelés"=TRUE) -> (w528:T5)
            n234 = Bundle By Name(cluster=w533, "Data"=w528) -> (w526:T4)
            n235 = Unbundle By Name(w526) -> ("Callback"=w527:string)
            n236 = call-poly "Enqueue Message.vi"("error in (no error)"=w521, "Message Data"=w526, "Message"=w527, "Message Queue"=w525) -> ("error out"=w537:errorcluster)  [unwired: 6 in, 1 out]
          }
          frame "DAQ Reset DO Port" {
            w569 = T4 {"Thread ID"=0, "Callback"="", "Data"=variant, "Error"={"status"=FALSE, "code"=0, "source"=""}}  # Message
            w572 = T5 {"Thread ID"=0.0, "Mérésszám"="", "Mérés/Utasítás"="", "Command"={"Parancs"="", "Paraméter 1"="", "Paraméter 2"="", "Paraméter 3"="", "Paraméter 4"="", "Paraméter 5"="", "Eredmény"=""}, "Min"="", "Max"="", "Aktív?"=FALSE, "Log?"=FALSE, "Kiértékelés"=FALSE, "Etalon 1 exp"=FALSE, "Etalon 2 exp"=FALSE, "Etalon 3 exp"=FALSE, "Etalon 4 exp"=FALSE, "Etalon 5 exp"=FALSE}  # Teszt cluster
            n237 = Variant To Data(error in=w568, type=w569, Variant=w565) -> (data=w563:T4, error out=w571:errorcluster)
            n238 = Unbundle By Name(w563) -> ("Data"=w570:variant)
            n239 = Variant To Data(error in=w571, type=w572, Variant=w570) -> (data=w566:T5, error out=w573:errorcluster)
            n240 = Unbundle By Name(w566) -> ("Command.Paraméter 3"=w561:string)
            n241 = Decimal String To Number(string=w561) -> (number=w560:i32)  [unwired: 2 in, 1 out]
            n242 = Unbundle By Name(w562) -> ("Engine"=w556:refnum<queue>, "NI Digital"=w555:refnum<queue>)
            n243 = call-poly "Enqueue Message.vi"("error in (no error)"=w573, "Message Data"=T2 {"PCIE-6321 OUT"={"Izolációs relé"=FALSE, "B oldal relé (nincs használva)"=FALSE, "48V relé"=FALSE, "Elszívás KI"=FALSE, "Bördelezés teszt"=FALSE, "Gyûrû megnyomás"=FALSE, "Termék rögzítés"=FALSE, "R mérés relé"=FALSE, "200mA relé"=FALSE, "NTC mérés relé"=FALSE, "Levegõ BE"=FALSE}} ("Digital output cluster"), "Message"="OUTPUT PortWrite", "Message Queue"=w555) -> ("error out"=w554:errorcluster)  [unwired: 6 in, 1 out]
            n244 = flat-sequence {
              tunnel: w554 -> [w574]
              tunnel: w560 -> [w575]
              tunnel: [w574] -> w552
              frame #0 {
                n245 = Wait (ms)(milliseconds to wait=w575) -> ()  [unwired: 1 out]
              }
            }
            n246 = Bundle By Name(cluster=w566, "Command.Eredmény"="DO Port Reseted", "Kiértékelés"=TRUE) -> (w559:T5)
            n247 = Bundle By Name(cluster=w563, "Data"=w559) -> (w557:T4)
            n248 = Unbundle By Name(w557) -> ("Callback"=w558:string)
            n249 = call-poly "Enqueue Message.vi"("error in (no error)"=w552, "Message Data"=w557, "Message"=w558, "Message Queue"=w556) -> ("error out"=w567:errorcluster)  [unwired: 6 in, 1 out]
          }
          frame "Write DO Single" {
            n250 = Variant To Data(error in=w587, type=cluster{i32, bool} {0, FALSE}, Variant=w585) -> (data=w578:cluster{i32, bool}, error out=w580:errorcluster)
            n251 = Unbundle(w578) -> (w576:i32, w577:bool)
            n252 = case shown="False" w577 {
              tunnel: ["OUTPUT BitSet" ("Message") "OUTPUT BitReset" ("Message")] -> w582
              frame True {
              }
              frame False {
              }
            }
            n253 = Greater Or Equal To 0?(x=w576) -> (x >= 0?=w583:bool)
            n254 = case shown="True" w583 {
              tunnel: w580 -> [w591 w594]
              tunnel: [w588 w594] -> w586
              tunnel: w581 -> [w593 _]
              tunnel: w576 -> [w590 _]
              tunnel: w582 -> [w589 _]
              frame True {
                # "Parancs végrehajtás"
                n255 = Unbundle By Name(w593) -> ("NI Digital"=w592:refnum<queue>)
                n256 = call-poly "Enqueue Message.vi"("error in (no error)"=w591, "Message Data"=w590, "Message"=w589, "Message Queue"=w592) -> ("error out"=w588:errorcluster)  [unwired: 6 in, 1 out]
              }
              frame False {
                # "Hibás csatorna név"
              }
            }
          }
          frame "Write AO" {
            n257 = Variant To Data(error in=w608, type=cluster{i32, dbl} {0, 0.0}, Variant=w606) -> (data=w597:cluster{i32, dbl}, error out=w600:errorcluster)
            n258 = Unbundle(w597) -> (w598:i32, w599:dbl)
            n259 = Greater Or Equal To 0?(x=w598) -> (x >= 0?=w604:bool)
            n260 = case shown="True" w604 {
              tunnel: w600 -> [w612 w615]
              tunnel: [w610 w615] -> w607
              tunnel: w602 -> [w614 _]
              tunnel: "OUTPUT Analog Write" ("Message") -> [w611 _]
              tunnel: w599 -> [_ _]
              tunnel: w597 -> [w609 _]
              frame True {
                # "Parancs végrehajtás"
                n261 = Unbundle By Name(w614) -> ("NI Analog"=w613:refnum<queue>)
                n262 = call-poly "Enqueue Message.vi"("error in (no error)"=w612, "Message Data"=w609, "Message"=w611, "Message Queue"=w613) -> ("error out"=w610:errorcluster)  [unwired: 6 in, 1 out]
              }
              frame False {
                # "Hibás csatorna név"
              }
            }
          }
          frame "Abort" {
            n263 = Flush Queue(queue=w618, error in (no error)=w619) -> (error out=w617:errorcluster)  [unwired: 2 out]
          }
          frame "Error" {
            n264 = Unbundle By Name(w626) -> ("UI"=w628:refnum<queue>)
            n265 = call-poly "Enqueue Message.vi"("error in (no error)"=w624, "Message Data"=w625, "Message"="Error", "Message Queue"=w628) -> ("error out"=w620:errorcluster)  [unwired: 6 in, 1 out]
            n266 = call-poly "Enqueue Message.vi"("Priority Message? (F)"=TRUE, "error in (no error)"=w624, "Message"="Initiate Stop", "Message Queue"=w631) -> ("error out"=w622:errorcluster)  [unwired: 6 in, 1 out]
            n267 = Merge Errors(w620, w622) -> (w621:errorcluster)
          }
          frame "Initiate Stop" {
            n268 = call-poly "Enqueue Message.vi"("Priority Message? (F)"=TRUE, "error in (no error)"=w633, "Message"="Program Stop", "Message Queue"=w636) -> ("error out"=w637:errorcluster)  [unwired: 6 in, 1 out]
          }
          frame "Program Stop" {
            n269 = Flush Queue(queue=w641, error in (no error)=w642) -> (error out=w639:errorcluster)  [unwired: 2 out]
          }
          frame Default {
            n270 = xnode "Error Ring"("parameter 0"=w643) -> ("error out"=w644:errorcluster)
          }
        }
      }
      frame True {
      }
    }
    n271 = call "Error Handler - Message Handling Loop.vi"("error in (no error)"=w12, "Message Queue"=w7) -> ("dup error in"=w13:errorcluster, "dup Message Queue"=w10:refnum<queue>)  [unwired: 8 in]
  }
  "error out" <- w6
  "Message Queue" <- w4
